vi "imaqio_Close.vi"(0 "Hardware Resource":T1, 5 "Abort before Close":bool) -> (15 "error out":errorcluster)   [LabVIEW 2017]
uses:
  <vilib>/LabVIEW Targets/FPGA/RIO/nirio_driverPrimitives.llb/_nirio_device_handleType.ctl
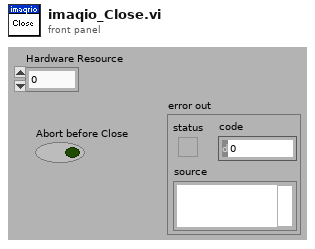
[diagram p1: front panel]
types:
  T1 = typedef "_nirio_device_handleType.ctl" = u32
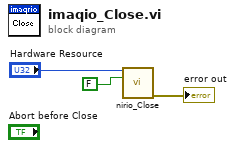
[diagram p0: block diagram]
diagram:
  n1 = call <vilib>:"nirio_Close.vi"("handle in"="Hardware Resource", "reset if last session (f)"=FALSE) -> ("error out"=→"error out":errorcluster)  [unwired: 13 out]
